vi "DEMO.vi"() -> ()   [LabVIEW 2012, in "Picture Box Tools.lvlib" / "Basic Shape.lvlib"]
uses:
  Basic Shape.lvlib
  Draw Para Custom Control.ctl
panel:
  in  "Draw Para":T1={"fill?(F)"=TRUE, "color(black)"=0, "pen"={"Width"=1, "Style"=enum."Solid"}}
  in  "Arrow":T2={"Line Len"=20, "Arrow dx"=-5, "Arrow dy"=5, "Line Angle"=0.0}
  in  "Start Pointx,y)":cluster{"x":i16, "y":i16} caption="Start Point(x,y)"
  out "Pic out 2":picture
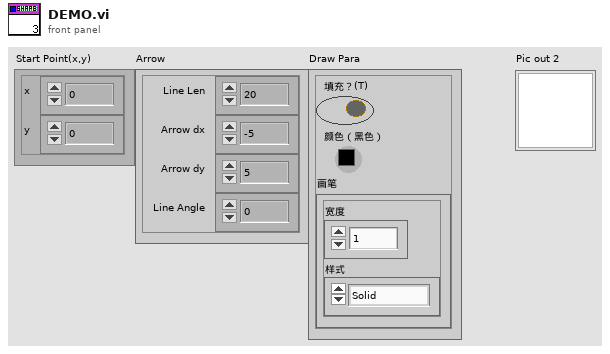
[diagram p1: front panel]
types:
  T1 = typedef "Picture Box Tools.lvlib/Basic Shape.lvlib/Draw Para Custom Control.ctl" = cluster{"fill?(F)":bool, "color(black)":u32, "pen":cluster{"Width":u16, "Style":enum32{"Solid", "Dash", "Dot", "DashDot", "DashDotDot"}}}
  T2 = cluster{"Line Len":i16, "Arrow dx":i16, "Arrow dy":i16, "Line Angle":dbl}
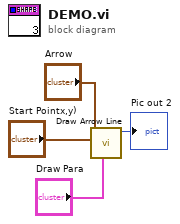
[diagram p0: block diagram]
diagram:
  n1 = call "Draw Arrow Line.vi"("Draw Para"="Draw Para", "Arrow"="Arrow", "Start Pointx,y)"="Start Pointx,y)") -> ("Pic out"=→"Pic out 2":picture)  [unwired: 7 in, 1 out]
